vi "Day 13 - Distress Signal.vi"() -> ()   [LabVIEW 2020, in "AoC 2022.lvlib"]
uses:
  AoC 2022.lvlib
  9e565855-789b-4a12-bcad-dab5c43d0287.vi
  9e565855-789b-4a12-bcad-dab5c43d0287.vi/4611cae3-c7be-41e2-9a5e-ea0ae78a7ced.vi
  9e565855-789b-4a12-bcad-dab5c43d0287.vi/4611cae3-c7be-41e2-9a5e-ea0ae78a7ced.vi/711a7bad-6791-4773-b8dd-6fbaf24e5b7c.vi
  9e565855-789b-4a12-bcad-dab5c43d0287.vi/4611cae3-c7be-41e2-9a5e-ea0ae78a7ced.vi/ab28192a-3d92-42da-8523-74871bf534c0.vi
  9e565855-789b-4a12-bcad-dab5c43d0287.vi/4611cae3-c7be-41e2-9a5e-ea0ae78a7ced.vi/d47d084a-d94a-47c5-b962-ca4ced011778.vi
  9e565855-789b-4a12-bcad-dab5c43d0287.vi/4611cae3-c7be-41e2-9a5e-ea0ae78a7ced.vi/0d0dd576-019e-4093-8822-9b4bde5edcbe.vi
  9e565855-789b-4a12-bcad-dab5c43d0287.vi/4611cae3-c7be-41e2-9a5e-ea0ae78a7ced.vi/148138b5-abcc-4d18-a1cb-fad94e4c517a.vi
  9e565855-789b-4a12-bcad-dab5c43d0287.vi/4611cae3-c7be-41e2-9a5e-ea0ae78a7ced.vi/46408cae-4ea5-4f15-ab36-8bc0fd18527a.vi
  9e565855-789b-4a12-bcad-dab5c43d0287.vi/4611cae3-c7be-41e2-9a5e-ea0ae78a7ced.vi/b1fbf645-60c9-4d68-8ae9-d3187fe658c2.vi
  9e565855-789b-4a12-bcad-dab5c43d0287.vi/4611cae3-c7be-41e2-9a5e-ea0ae78a7ced.vi/5179999f-faab-4e10-925a-f43c3f28d8d8.vi
  9e565855-789b-4a12-bcad-dab5c43d0287.vi/4611cae3-c7be-41e2-9a5e-ea0ae78a7ced.vi/14adcb6d-7f20-40e2-b0f4-539fd4458acc.vi
  private/Sorter/Less Than.vi
panel:
  out "Compared Items out":string
  in  "Puzzle Input":string="[1,1,3,1,1]\n[1,1,5,1,1]\n\n[[1],[2,3,4]]\n[[1],4]\n\n[9]\n[[8,7,6]]\n\n[[4,4],4,4]\n[[4,4],4,4,4]\n\n[7,7,7,7]\n[7,7,7]\n\n[]\n[3]\n\n[[[]]]\n[[]]\n\n[1,[2,[3,[4,[5,6,7]]]],8,9]\n[1,[2,[3,[4,[5,6,0]]]],8,9]"
  out "Puzzle Part-2 Answer":string
  out "Puzzle Answer":string
  # "Press Ctrl+M & Enter the Puzzle Input and run the VI"
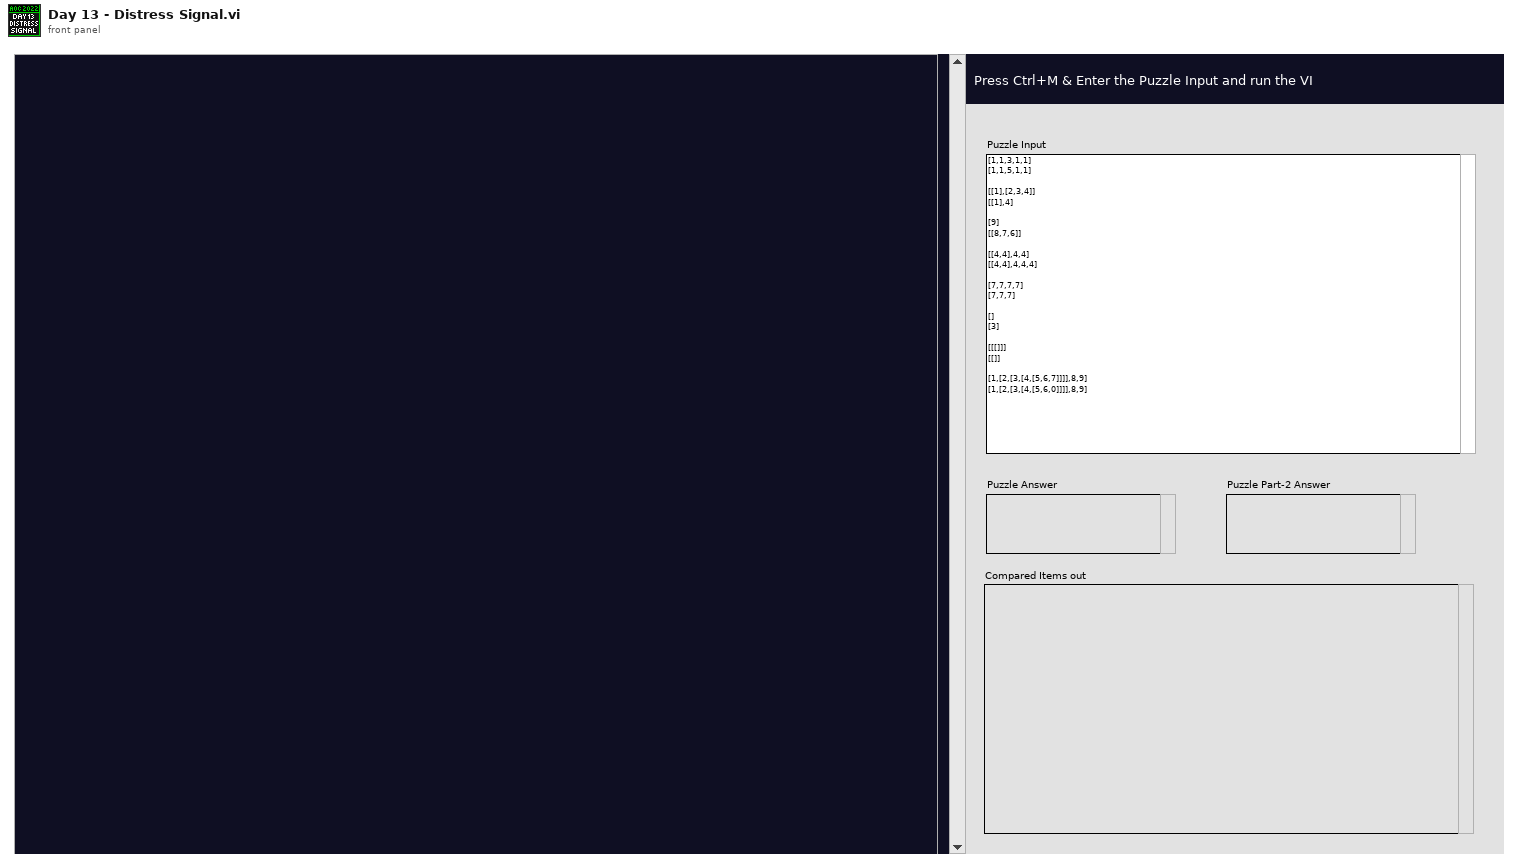
[diagram p1: front panel]
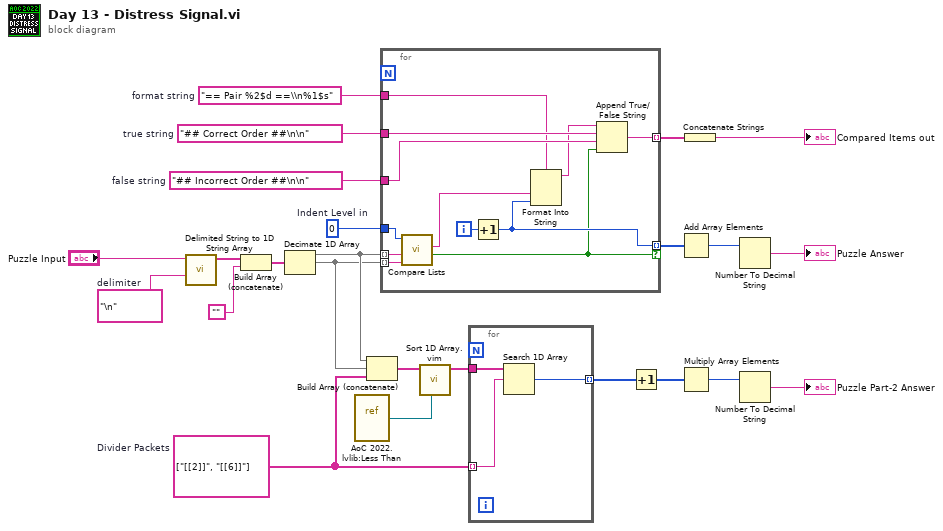
[diagram p0: block diagram]
diagram:
  w4 = string[] ["[[2]]", "[[6]]"]  # Divider Packets
  w10 = "== Pair %2$d ==\\n%1$s"  # format string
  w12 = 0  # Indent Level in
  w13 = "## Incorrect Order ##\n\n"  # false string
  w14 = "## Correct Order ##\n\n"  # true string
  w22 = "\n"  # delimiter
  n1 = call <vilib>:"Delimited String to 1D String Array.vi"("delimiter"=w22, "delimited string"="Puzzle Input") -> ("string array"=w20:string[])  [unwired: 9 in]
  n2 = Build Array (concatenate)(w20, "") -> (w19:string[])
  n3 = Decimate 1D Array(w19) -> (w9:string[], w8:string[])  [unwired: 1 out]
  n4 = vi-ref "AoC 2022.lvlib:Less Than.vi"() -> (w6:refnum<vi>)
  n5 = Build Array (concatenate)(w9, w8, w4) -> (w7:string[])
  n6 = for {
    tunnel: w9 -> [w36] mode=indexing
    tunnel: w8 -> [w35] mode=indexing
    tunnel: [w28] -> w17 mode=indexing if=w25
    tunnel: [w34] -> w15 mode=indexing
    tunnel: w14 -> [w33]
    tunnel: w13 -> [w32]
    tunnel: w12 -> [w31]
    tunnel: w10 -> [w26]
    i -> [w29]
    n7 = call "Compare Lists.vi"("Right List"=w35, "Left List"=w36, "Indent Level in"=w31) -> ("In Right Order ?"=w25:bool, "Compared Items out"=w30:string)  [unwired: 1 in, 2 out]
    n8 = Increment(x=w29) -> (x+1=w28:i32)
    n9 = Format Into String(format string=w26, w30, w28) -> (resulting string=w27:string)  [unwired: 2 in, 1 out]
    n10 = Append True/False String(1:w25, 2:w32, 3:w33, 4:w27) -> (0:w34:string)
  }
  n11 = call "Sort 1D Array.vim"("less function (built-in <)"=w6, "unsorted array"=w7) -> ("sorted array"=w5:string[])  [unwired: 9 in]
  n12 = for {
    tunnel: w5 -> [w39]
    tunnel: w4 -> [w38] mode=indexing
    tunnel: [w37] -> w3 mode=indexing
    n13 = Search 1D Array(1D array=w39, element=w38) -> (index of element=w37:i32)  [unwired: 1 in]
  }
  n14 = Increment(x=w3) -> (x+1=w2:i32[])
  n15 = Add Array Elements(numeric array=w17) -> (sum=w16:i32)
  n16 = Multiply Array Elements(1:w2) -> (0:w1:i32)
  n17 = Concatenate Strings(w15) -> (→"Compared Items out":string)
  n18 = Number To Decimal String(number=w16) -> (decimal integer string=→"Puzzle Answer":string)  [unwired: 1 in]
  n19 = Number To Decimal String(number=w1) -> (decimal integer string=→"Puzzle Part-2 Answer":string)  [unwired: 1 in]
